vi "writeToXML.vi"(8 "error in (no error)":errorcluster, 10 "ClassLabel":string, 11 "PointingFileCommands in":refnum<class "PointingFileCommands.lvclass">) -> (0 "error out":errorcluster, 2 "XML out":string, 3 "PointingFileCommands out":refnum<class "PointingFileCommands.lvclass">)   [LabVIEW 2014, in "TCSDataDefinitions.lvlib" / "TCSCommand.lvlib" / "PointingFileCommands.lvlib" / "PointingFileCommands.lvclass"]
uses:
  PointingFileCommands.lvclass
  TCSTcsCommand/TCSTcsCommand.lvclass
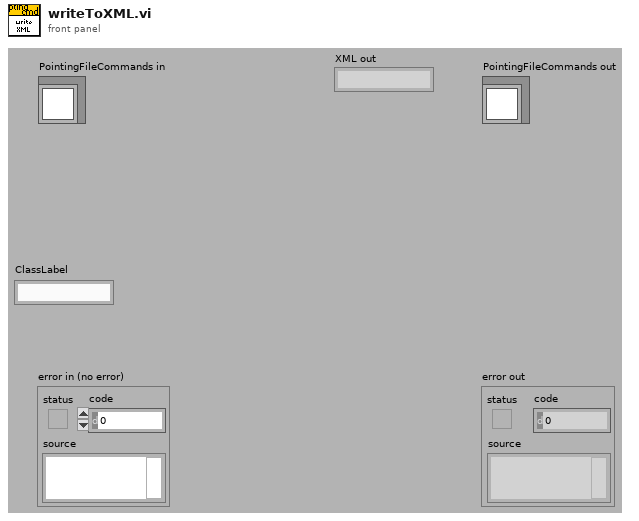
[diagram p1: front panel]
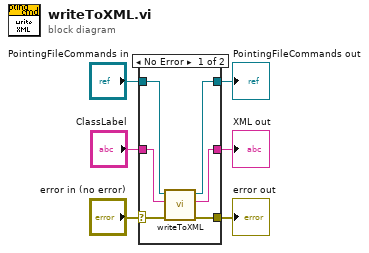
[diagram p0: block diagram]
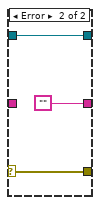
[diagram p2: hidden frame]
diagram:
  n1 = case shown="No Error" "error in (no error)" {
    selector: "error in (no error)" -> [w8 w15]
    tunnel: [w7 w15] -> w5
    tunnel: [w11 w14] -> w3
    tunnel: "PointingFileCommands in" -> [w12 w14]
    tunnel: "ClassLabel" -> [w10 _]
    tunnel: [w9 ""] -> w1
    frame No Error {
      n2 = call-parent "writeToXML.vi"("error in (no error)"=w8, "ClassLabel"=w10, "TCSTcsCommand in"=w12) -> ("error out"=w7:errorcluster, "XML out"=w9:string, "TCSTcsCommand out"=w11:refnum<class "PointingFileCommands.lvclass">)  [unwired: 6 in]
    }
    frame Error {
    }
  }
  "error out" <- w5
  "PointingFileCommands out" <- w3
  "XML out" <- w1
